vi "Get Type Enum.vi"(8 "error in (no error)":errorcluster, 11 "EquipmentVariant in":refnum<class "EquipmentVariant.lvclass">) -> (0 "error out":errorcluster, 2 "Type":T1=enum."Instrument", 3 "EquipmentVariant out":refnum<class "EquipmentVariant.lvclass">)   [LabVIEW 2020, in "EquipmentVariant.lvclass"]
uses:
  EquipmentVariant.lvclass
  home/jki/EnumeratedVariant/EnumeratedVariant/EnumeratedVariant.lvclass
  Type Enum.ctl
  EnumeratedVariant/EnumeratedVariant.lvclass/EnumeratedVariant.ctl
  290bd5ce-6024-3fef-d031-90816207e13f.vi
  EnumeratedVariant/Read VEnum.vi
  EquipmentVariant.lvclass/EquipmentVariant.ctl
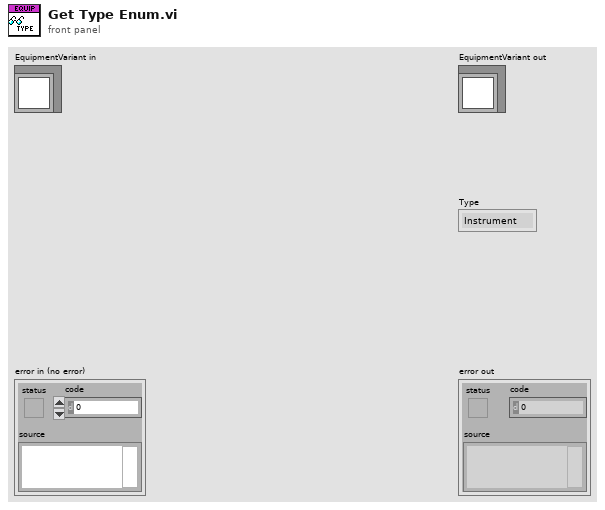
[diagram p1: front panel]
types:
  T1 = typedef "EquipmentVariant.lvclass/Type Enum.ctl" = enum16{"Robot", "Pump", "Instrument"}
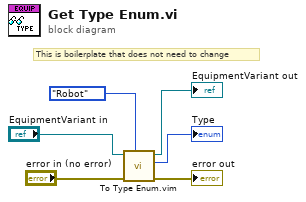
[diagram p0: block diagram]
diagram:
  # "This is boilerplate that does not need to change"
  n1 = call "To Type Enum.vim"("type"=Type_Enum."Robot" ("Type"), "error in (no error)"="error in (no error)", "EnumeratedVariant in"="EquipmentVariant in") -> ("error out"=→"error out":errorcluster, "Enum"=→"Type":T1, "EnumeratedVariant out"=→"EquipmentVariant out":refnum<class "EquipmentVariant.lvclass">)  [unwired: 6 in]
